vi "InfoGui.vi"(6 "Button texts":T1[](array[typedef])=[enum."OK", enum."Cancel"], 7 "_onebutton(F)":bool caption="one button (F)", 9 "_Arg":variant[](array[variant]), 10 "_Msg":T1) -> (2 "ok":bool)   [LabVIEW 2016]
uses:
  Tools/Translator/Translator.Message.ctl
  InfoGui.Action.ctl
  Tools/Translator/Translator.FormatMessage.vi
  Tools/Translator/Translator.Global.vi
panel:
  out "_loop":i32(ring)=4
  in  "CancelButton":bool
  out "Message":string
  in  "OKButton":bool
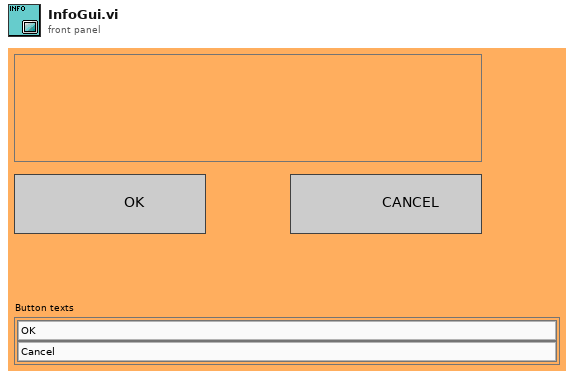
[diagram p1: front panel]
types:
  T1 = typedef "Translator.Message.ctl" = enum16{"-", "Event confirmed", "Log out", "Log in", "Shutdown", "Cancel", "Start", "Continue", "Stop", "On", "Off", "OK", "NOK", "NOK %s", "This", "Prev", "Home", "Work", "In progress...", "Missing", "Empty", "Hardware failure", "Initial", "Error %d >> %s", "Error %d >> %s >> %s", "Starting %s", "Quitting %s", "Configured", "Initializing", "Quitting", "Loading", "Running %s", "Stopped", "Summary", "Do you want to continue?", "Do you want to exit?", "Log out?", "System", "All", "IDLE", "Translating...%s", "Not found", "Alarm %s", "Run", "Skip", "Abort", "Repeat", "Please wait...", "Database disconnected", "Login to database successful", "Login to database failed: %d; %s", "Get process step data for %s", "Changeover off", "Changeover into %s", "Product %s | %s found in cache with status %d at previous station", "Product %s | %s found in database with status %d at previous station", "Product %s | %s not found in cache at previous station", "Product %s | %s not found in database at previous station", "Product %s | %s found in cache with status %d at this station (%d repetion)", "Product %s | %s found in database with status %d at this station (%d repetition)", "Product %s | %s not found in cache at this station", "Product %s | %s not found in database at this station", "Product %s | %s found in cache for component %s | %s", "Product %s | %s found in database for component %s | %s", "Product not found in cache for component %s | %s", "Product not found in database for component %s | %s", "Product %s | %s connected with component %s | %s (cache)", "Product %s | %s connected with component %s | %s (database)", "New data for %s | %s (cache)", "New data for %s | %s (database)", "File %s moved (cache)", "File %s deleted (cache)", "Msg %d >> %s", "PLC LifeBit Failure", "Reconnecting DB", "Reconnecting PLC", "Free disk space is below 1GB - contact technician", "Unable to check product status", "Product %s SN %s checked in DB"}
  T2 = typedef "InfoGui.Action.ctl" = enum32{"idle", "constructor", "destructor", "--- InfoGUI ---"}
  T3 = typedef "LVPositionTypeDef.ctl" = cluster{"Left":i32, "Top":i32}
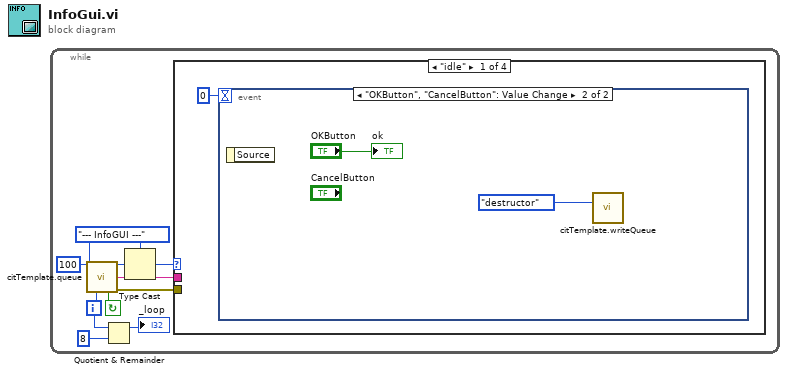
[diagram p0: block diagram]
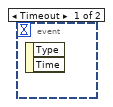
[diagram p2: hidden frame]
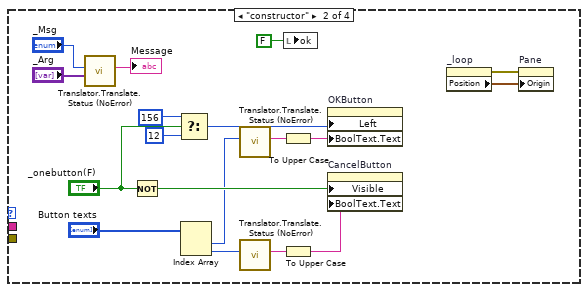
[diagram p3: hidden frame]
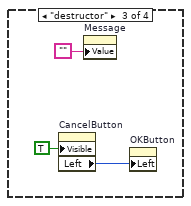
[diagram p4: hidden frame]
diagram:
  n1 = while {
    i -> [w1]
    stop <- w10 continue-if-true
    w4 = InfoGui.Action."--- InfoGUI ---" ("Action")
    n2 = call "citTemplate.queue.vi"("ms timeout (250 ms)"=100, "event enum"=w4, "iteration (-1)"=w1) -> ("event out"=w8:u32, "(flatten) data out"=w5:string, "continue"=w10:bool, "error out"=w6:errorcluster)  [unwired: 2 in, 7 out]
    n3 = Quotient & Remainder(x=w1, y=8) -> (x-y*floor(x/y)=→"_loop":i32)  [unwired: 1 out]
    n4 = Type Cast(type=w4, x=w8) -> (*(type *) &x=w7:T2)
    n5 = case shown="\"idle\"" w7 {
      tunnel: w6 -> [_ _ _ _]
      tunnel: w5 -> [_ _ _ _]
      frame "idle" {
        n6 = event shown="[1] \"OKButton\", \"CancelButton\": Value Change" {
          selector: _ -> [_ _]
          dyn-events: _ -> [_ _]
          timeout: 0 -> [_ _]
          event Timeout {
            n7 = event-data() -> ()  [unwired: 3 out]
          }
          event "OKButton", "CancelButton": Value Change {
            n8 = event-data() -> ()  [unwired: 2 out]
            n9 = call "citTemplate.writeQueue.vi"("event in (if not connected:all statemachine with data event)"=InfoGui.Action."destructor" ("Action")) -> ()  [unwired: 14 in, 1 out]
            "ok" <- "OKButton"
          }
        }
      }
      frame "constructor" {
        n10 = call "Translator.Translate.Status (NoError).vi"("Arguments"="_Arg", "msg"="_Msg") -> ("Translated Msg"=→"Message":string)  [unwired: 9 in]
        n11 = Not(x="_onebutton(F)") -> (.not. x?=w30:bool)
        n12 = Select(t=156 ("Position:Left"), s="_onebutton(F)", f=12) -> (s? t:f=w21:i32)
        n13 = Index Array(array="Button texts") -> (element #1=w18:T1, element #2=w17:T1)  [unwired: 2 in]
        n14 = call "Translator.Translate.Status (NoError).vi"("msg"=w18) -> ("Translated Msg"=w19:string)  [unwired: 10 in]
        n15 = call "Translator.Translate.Status (NoError).vi"("msg"=w17) -> ("Translated Msg"=w16:string)  [unwired: 10 in]
        n16 = To Upper Case(1:w19) -> (0:w15:string)
        n17 = To Upper Case(1:w16) -> (0:w14:string)
        n18 = local write "ok"(FALSE ("_b_ok")) -> ()
        n19 = property on="OKButton" class="Bool"("Left"=w21, "BoolText.Text"=w15) -> ()  [unwired: 2 in, 2 out]
        n20 = property on="CancelButton" class="Bool"("Visible"=w30, "BoolText.Text"=w14) -> ()  [unwired: 2 in, 2 out]
        n21 = property on="_loop" class="Ring (strict)"() -> (error out=w22:errorcluster, "Position"=w23:T3)  [unwired: 2 in, 1 out]
        n22 = property on="Pane" class="Pane"(error in=w22, "Origin"=w23) -> ()  [unwired: 1 in, 2 out]
      }
      frame "destructor" {
        n23 = property on="CancelButton" class="Bool"("Visible"=TRUE) -> ("Left"=w32:i32)  [unwired: 2 in, 2 out]
        n24 = property on="Message" class="Str"("Value"="") -> ()  [unwired: 2 in, 2 out]
        n25 = property on="OKButton" class="Bool"("Left"=w32) -> ()  [unwired: 2 in, 2 out]
      }
      frame "--- InfoGUI ---" {
      }
    }
  }
